vi "Close.vi"(8 "error in":errorcluster, 11 "Thermometer DAQmx TC Cont CFG in":refnum<class "Thermometer DAQmx TC Cont CFG.lvclass">) -> (0 "error out":errorcluster, 3 "Thermometer DAQmx TC Cont CFG out":refnum<class "Thermometer DAQmx TC Cont CFG.lvclass">)   [LabVIEW 2024, in "Thermometer DAQmx TC Cont CFG.lvclass"]
uses:
  Thermometer DAQmx TC Cont CFG.lvclass
  Thermometer DAQmx TC Cont CFG.lvclass/Thermometer DAQmx TC Cont CFG.ctl
  DAQmx Base CFG/DAQmx Base CFG.lvclass
  Buffers/Buffer Lossless DBL/Buffer Lossless DBL.lvclass
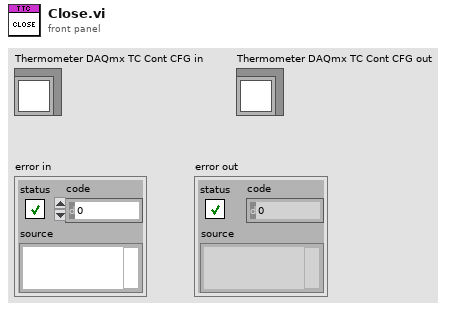
[diagram p1: front panel]
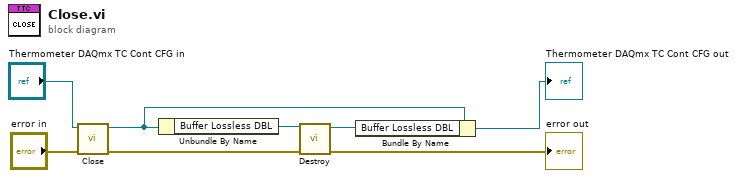
[diagram p0: block diagram]
diagram:
  n1 = call-parent "Close.vi"("error in"="error in", "DAQmx Base CFG in"="Thermometer DAQmx TC Cont CFG in") -> ("error out"=w5:errorcluster, "DAQmx Base CFG out"=w2:refnum<class "Thermometer DAQmx TC Cont CFG.lvclass">)  [unwired: 8 in]
  n2 = Unbundle By Name(w2) -> ("Buffer Lossless DBL"=w6:refnum<class "Buffer Lossless DBL.lvclass">)
  n3 = call "Destroy.vi"("error in"=w5, "Buffer Lossless DBL in"=w6) -> ("error out"=→"error out":errorcluster, "Buffer Lossless DBL out"=w3:refnum<class "Buffer Lossless DBL.lvclass">)  [unwired: 8 in]
  n4 = Bundle By Name(cluster=w2, "Buffer Lossless DBL"=w3) -> (→"Thermometer DAQmx TC Cont CFG out":refnum<class "Thermometer DAQmx TC Cont CFG.lvclass">)
